vi "tutorial-VISAWriteRead3.vi"() -> ()   [LabVIEW 2020]
panel:
  out "read buffer":string
  in  "write buffer":string
  in  "VISA resource name":refnum<visa-resource-name>
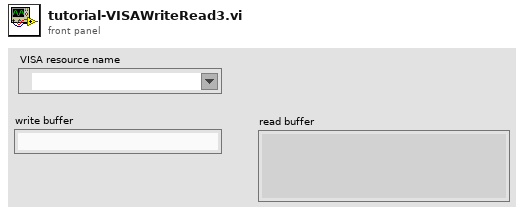
[diagram p1: front panel]
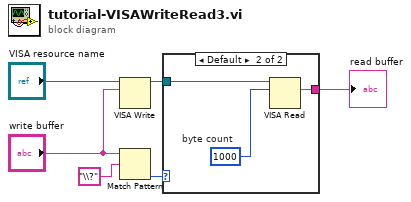
[diagram p0: block diagram]
diagram:
  n1 = VISA Write(VISA resource name="VISA resource name", write buffer="write buffer") -> (VISA resource name out=w5:refnum<visa-resource-name>)  [unwired: 1 in, 2 out]
  n2 = Match Pattern(string="write buffer", regular expression="\\?") -> (offset past match=w1:i32)  [unwired: 1 in, 3 out]
  n3 = case shown="Default" w1 {
    tunnel: w5 -> [_ w9]
    tunnel: [_ w7] -> w2
    frame -1 {
    }
    frame Default {
      w8 = u32 1000  # byte count
      n4 = VISA Read(VISA resource name=w9, byte count=w8) -> (read buffer=w7:string)  [unwired: 1 in, 3 out]
    }
  }
  "read buffer" <- w2
